vi "Update controls.vi"(8 "error in (no error)":errorcluster, 10 "New control values":variant, 11 "PS Control Actor in":refnum<class "PS Control Actor.lvclass">) -> (0 "error out":errorcluster, 3 "PS Control Actor out":refnum<class "PS Control Actor.lvclass">)   [LabVIEW 2025, in "PS Control Actor.lvlib" / "PS Control Actor.lvclass"]
doc: "Author: Scott Hannahs <sth@magnet.fsu.edu>\n\nThis software is licensed for use under the “MIT License\"\nCopyright (c) 2025 Scott Hannahs, sth@sth@magnet.sthnet.net\n\nPermission is hereby granted, free of charge, to any person obtaining a copy of this software and associated documentation files (the \"Software\"), to deal in the Software without restriction, including without limitation the rights to use, copy, modify, merge, publish, distribute, sublicense, and/or sell copies of the Software, and to permit persons to whom the Software is furnished to do so, subject to the following conditions: The above copyright notice and this permission notice shall be included in all copies or substantial portions of the Software.\n\nTHE SOFTWARE IS PROVIDED \"AS IS\", WITHOUT WARRANTY OF ANY KIND, EXPRESS OR IMPLIED, INCLUDING BUT NOT LIMITED TO THE WARRANTIES OF MERCHANTABILITY, FITNESS FOR A PARTICULAR PURPOSE AND NONINFRINGEMENT. IN NO EVENT SHALL THE AUTHORS OR COPYRIGHT HOLDERS BE LIABLE FOR ANY CLAIM, DAMAGES OR OTHER LIABILITY, WHETHER IN AN ACTION OF CONTRACT, TORT OR OTHERWISE, ARISING FROM, OUT OF OR IN CONNECTION WITH THE SOFTWARE OR THE USE OR OTHER DEALINGS IN THE SOFTWARE."
uses:
  PS Control Actor.lvclass
  PS Control Actor.lvclass/PS Control Actor.ctl
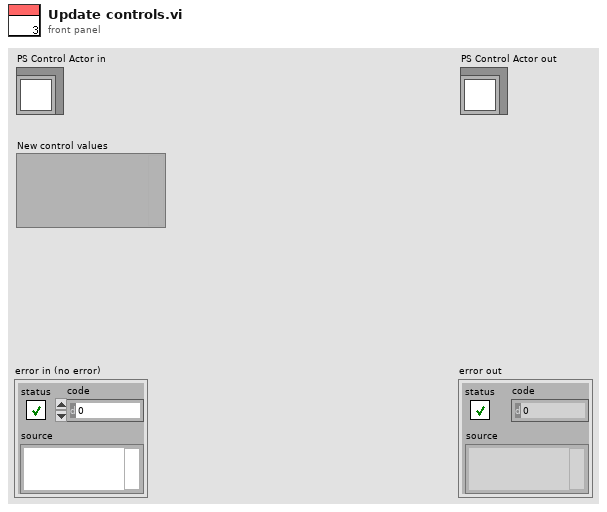
[diagram p1: front panel]
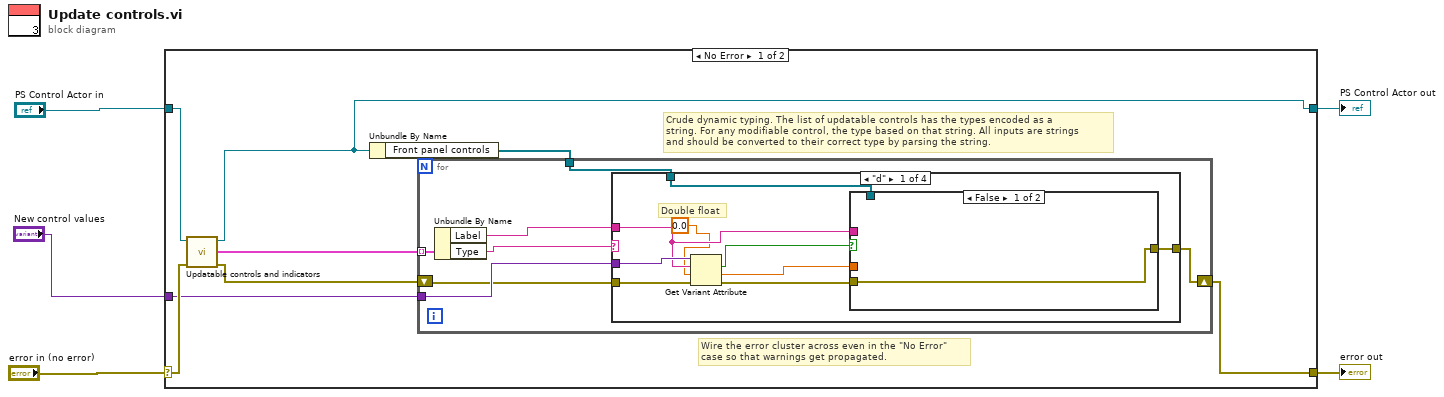
[diagram p0: block diagram]
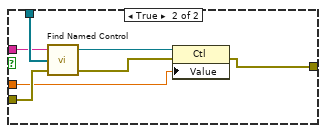
[diagram p2: hidden frame]
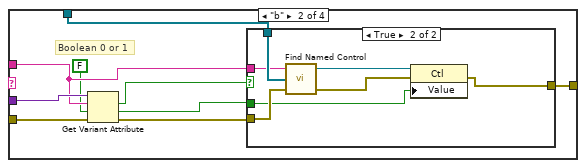
[diagram p3: hidden frame]
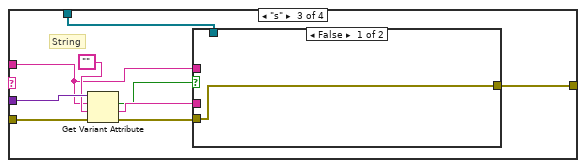
[diagram p5: hidden frame]
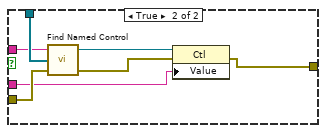
[diagram p6: hidden frame]
diagram:
  n1 = case shown="No Error" "error in (no error)" {
    selector: "error in (no error)" -> [w11 w74]
    tunnel: [w12 w74] -> w4
    tunnel: [w7 w73] -> w2
    tunnel: "PS Control Actor in" -> [w8 w73]
    tunnel: "New control values" -> [w6 _]
    frame No Error {
      # "Crude dynamic typing. The list of updatable controls has the types encoded as a\nstring. For any modifiable control, the type based on that string. All inputs are strings\nand should be converted to their correct type by parsing the string."
      # "Wire the error cluster across even in the \"No Error\"\ncase so that warnings get propagated."
      n2 = call-dynamic "Updatable controls and indicators.vi"("error in (no error)"=w11, "PS Control Actor in"=w8) -> ("error out"=w10:errorcluster, "Control type list"=w9:cluster{"Label":string, "Type":string}[], "PS Control Actor out"=w7:refnum<class "PS Control Actor.lvclass">)  [unwired: 7 in]
      n3 = Unbundle By Name(w7) -> ("Front panel controls"=w13:refnum<vi>[])
      n4 = for {
        tunnel: w13 -> [w20]
        tunnel: w9 -> [w19] mode=indexing
        tunnel: w6 -> [w18]
        shift-right: [w15] -> w12
        shift-left: w10 -> [w14]
        n5 = Unbundle By Name(w19) -> ("Label"=w17:string, "Type"=w16:string)
        n6 = case shown="\"d\"" w16 {
          tunnel: w20 -> [w26 w43 w58 _]
          tunnel: w18 -> [w29 w46 w63 _]
          tunnel: w17 -> [w23 w40 w55 _]
          tunnel: w14 -> [w28 w45 w62 w72]
          tunnel: [w25 w42 w57 w72] -> w15
          frame "d" {
            # "Double float"
            n7 = Get Variant Attribute(Variant=w29, name=w23, default value (empty Variant)=0.0, error in=w28) -> (found=w24:bool, value=w21:dbl, error out=w27:errorcluster)  [unwired: 1 out]
            n8 = case shown="False" w24 {
              tunnel: w26 -> [_ w37]
              tunnel: w27 -> [w30 w34]
              tunnel: w21 -> [_ w33]
              tunnel: [w30 w32] -> w25
              tunnel: w23 -> [_ w31]
              frame False {
              }
              frame True {
                n9 = call "Find Named Control.vi"("error in"=w34, "All Controls"=w37, "Control Name"=w31) -> ("error out"=w35:errorcluster, "Ctl Refnum"=w36:refnum<vi>)  [unwired: 1 out]
                n10 = property class="Ctl"(reference=w36, error in=w35, "Value"=w33) -> (error out=w32:errorcluster)  [unwired: 1 out]
              }
            }
          }
          frame "b" {
            # "Boolean 0 or 1"
            n11 = Get Variant Attribute(Variant=w46, name=w40, default value (empty Variant)=FALSE, error in=w45) -> (found=w41:bool, value=w38:bool, error out=w44:errorcluster)  [unwired: 1 out]
            n12 = case shown="True" w41 {
              tunnel: w43 -> [_ w54]
              tunnel: w44 -> [w47 w51]
              tunnel: w38 -> [_ w50]
              tunnel: [w47 w49] -> w42
              tunnel: w40 -> [_ w48]
              frame False {
              }
              frame True {
                n13 = call "Find Named Control.vi"("error in"=w51, "All Controls"=w54, "Control Name"=w48) -> ("error out"=w52:errorcluster, "Ctl Refnum"=w53:refnum<vi>)  [unwired: 1 out]
                n14 = property class="Ctl"(reference=w53, error in=w52, "Value"=w50) -> (error out=w49:errorcluster)  [unwired: 1 out]
              }
            }
          }
          frame "s" {
            # "String"
            n15 = Get Variant Attribute(Variant=w63, name=w55, default value (empty Variant)="", error in=w62) -> (found=w56:bool, value=w60:string, error out=w61:errorcluster)  [unwired: 1 out]
            n16 = case shown="False" w56 {
              tunnel: w58 -> [_ w71]
              tunnel: w61 -> [w64 w68]
              tunnel: w60 -> [_ w67]
              tunnel: [w64 w66] -> w57
              tunnel: w55 -> [_ w65]
              frame False {
              }
              frame True {
                n17 = call "Find Named Control.vi"("error in"=w68, "All Controls"=w71, "Control Name"=w65) -> ("error out"=w69:errorcluster, "Ctl Refnum"=w70:refnum<vi>)  [unwired: 1 out]
                n18 = property class="Ctl"(reference=w70, error in=w69, "Value"=w67) -> (error out=w66:errorcluster)  [unwired: 1 out]
              }
            }
          }
          frame Default {
          }
        }
      }
    }
    frame Error {
    }
  }
  "error out" <- w4
  "PS Control Actor out" <- w2
